vi "reset.vi"(0 "Interface in":T1, 11 "error in (no error)":errorcluster) -> (4 "Interface out":T1, 15 "error out":errorcluster)   [LabVIEW 2017, in "BuckBoostInterface.lvlib"]
uses:
  BuckBoostInterface.lvlib
  Interface.ctl
  <instrlib>/_niInstr/Instruction Framework/v1/Host/Instruction Target/niInstr Instruction Target v1 Host.lvclass
  <instrlib>/_niInstr/Instruction Framework/v1/Host/Instruction Framework Context/niInstr Instruction Framework Context v1 Host.lvclass
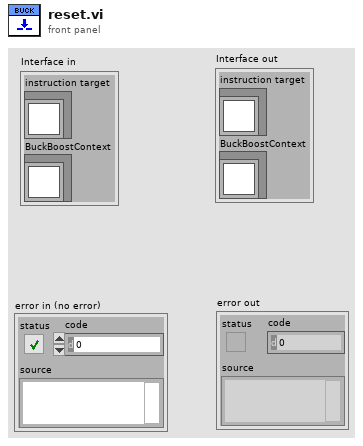
[diagram p1: front panel]
types:
  T1 = typedef "BuckBoostInterface.lvlib/Interface.ctl" = cluster{"instruction target":refnum<class "niInstr Instruction Target v1 Host.lvclass">, "BuckBoostContext":refnum<class "niInstr Instruction Framework Context v1 Host.lvclass">}
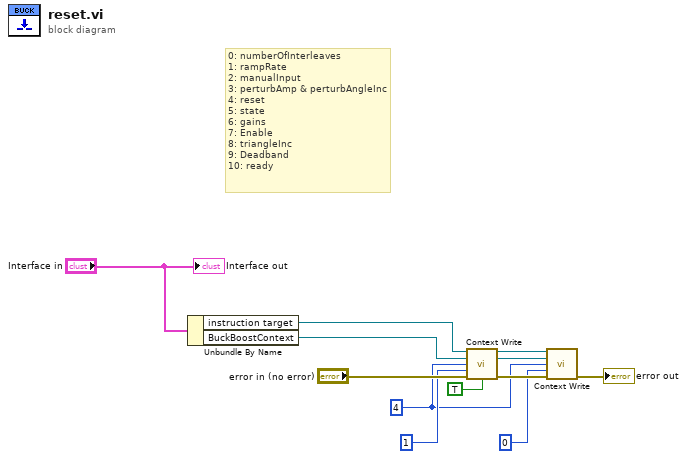
[diagram p0: block diagram]
diagram:
  w2 = u64 4 ("address")
  # "0: numberOfInterleaves\n1: rampRate\n2: manualInput\n3: perturbAmp & perturbAngleInc\n4: reset\n5: state\n6: gains\n7: Enable\n8: triangleInc\n9: Deadband\n10: ready"
  n1 = Unbundle By Name("Interface in") -> ("instruction target"=w10:refnum<class "niInstr Instruction Target v1 Host.lvclass">, "BuckBoostContext"=w9:refnum<class "niInstr Instruction Framework Context v1 Host.lvclass">)
  n2 = call <instrlib>:"Context Write.vi"("instruction target in"=w10, "context in"=w9, "address"=w2, "data"=u64 1, "error in"="error in (no error)", "wait until committed (T)"=TRUE) -> ("instruction target out"=w6:refnum<class "niInstr Instruction Target v1 Host.lvclass">, "context out"=w3:refnum<class "niInstr Instruction Framework Context v1 Host.lvclass">, "error out"=w5:errorcluster)  [unwired: 7 in]
  n3 = call <instrlib>:"Context Write.vi"("instruction target in"=w6, "context in"=w3, "address"=w2, "data"=u64 0, "error in"=w5) -> ("error out"=→"error out":errorcluster)  [unwired: 8 in, 2 out]
  "Interface out" <- "Interface in"
